vi "Get Version.vi"(8 "error in":errorcluster, 9 "index":i32, 11 "Builder in":refnum<class "Builder.lvclass">) -> (0 "error out":errorcluster, 1 "Build Version (String)":string, 2 "Build Version":T1, 3 "Builder out":refnum<class "Builder.lvclass">)   [LabVIEW 2021, in "App-Builder Library.lvlib" / "Builder.lvclass"]
uses:
  Builder.lvclass
  <vilib>/AppBuilder/AB_API_Simple/Build Specification Version.ctl
  Builder.lvclass/Builder.ctl
  <vilib>/AppBuilder/AB_API_Simple/Get Build Specification Version (path).vi
  <vilib>/AppBuilder/AB_API_Simple/NI_App_Builder_API.lvlib
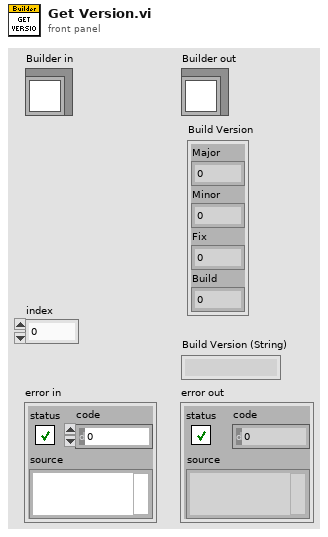
[diagram p1: front panel]
types:
  T1 = typedef "NI_App_Builder_API.lvlib/Build Specification Version.ctl" = cluster{"Major":u16, "Minor":u16, "Fix":u16, "Build":u16}
  T2 = typedef "App-Builder Library.lvlib/Builder.lvclass/Build specification.ctl" = cluster{"target name":string, "Build specification":string, "Project Path":path, "Build Object type":T3}
  T3 = typedef "App-Builder Library.lvlib/Builder.lvclass/Build object type.ctl" = enum16{"EXE", "RT EXE", "Deployable Packed"}
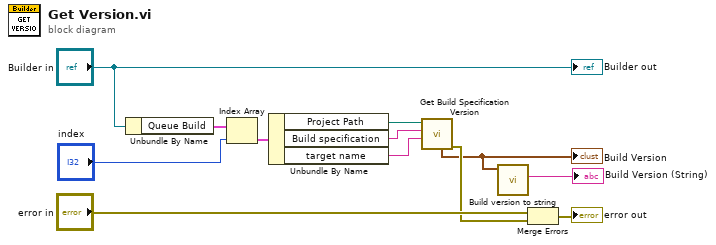
[diagram p0: block diagram]
diagram:
  n1 = Unbundle By Name("Builder in") -> ("Queue Build"=w5:T2[])
  n2 = Index Array(array=w5, index="index") -> (element=w4:T2)
  n3 = Unbundle By Name(w4) -> ("Project Path"=w8:path, "Build specification"=w7:string, "target name"=w6:string)
  n4 = call-poly <vilib>:"Get Build Specification Version.vi"("Name of target (My Computer)"=w6, "Name of build specification"=w7, "Path to project"=w8) -> ("error out"=w9:errorcluster, "Build Specification Version"=w2:T1)  [unwired: 7 in]
  "Build Version" <- w2
  n5 = call "Build version to string.vi"("Build Version"=w2) -> ("Build Version (String)"=→"Build Version (String)":string)  [unwired: 10 in]
  n6 = Merge Errors("error in", w9) -> (→"error out":errorcluster)
  "Builder out" <- "Builder in"
